vi "LVFunction_Imop_HAS file_GetInformation.vi"(0 "HAS file path":path, 11 "error in (no error)":errorcluster) -> (6 "HAS file information":T1 {"Source wavelength (nm)" format="%#_2g"}, 15 "error out":errorcluster)   [LabVIEW 2020]
doc: "Get informations from .has file.\n\n--------------------------------------------------------------------------------\n\n<B>has_file_pathIn</B> : Absolute path to the .has file.\n\n<B>has_file_pathOut</B> : Absolute path to the .has file.\n\n<B>haso_model</B> : Haso Sensor model.\n\n<B>haso_serial_number</B> : Haso Serial number.\n\n<B>revision</B> : Revision number.\n\n<B>size</B> : HasoData dimension (subpupil number)\n\n<B>step</B> : HasoData sampling step (um).\n\n<B>time_stamp</B> : Timestamp.\n\n<B>comments</B> : Comments\n\n<B>session_name</B> : Session name.\n\n<B>wavelength_nm</B> : Source wavelength (nm).\n\n<B>lower_calibration_wl</B> : Lower calibration wavelength (nm).\n\n<B>upper_calibration_wl</B> : Upper calibration wavelength (nm).\n\n<B>ErrorIn</B> : Error\n\n<B>ErrorOut</B> : Error"
uses:
  Controls/HAS File information.ctl
  Controls/General dimensions definition.ctl
  Controls/Point2D.ctl
  Controls/Point2Df.ctl
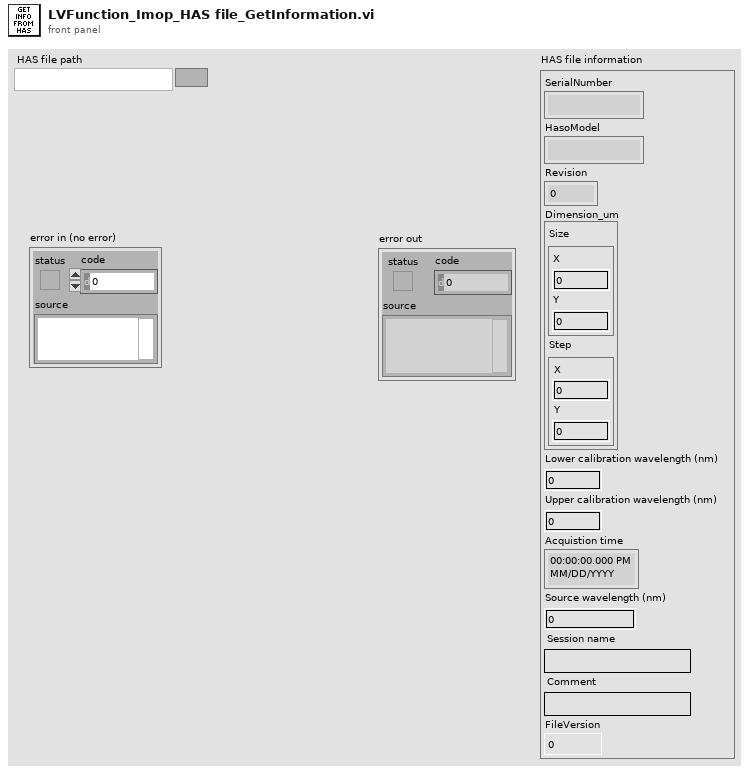
[diagram p1: front panel]
types:
  T1 = typedef "HAS File information.ctl" = cluster{"SerialNumber":string, "HasoModel":string, "Revision":u32, "Dimension_um":T2, "Lower calibration wavelength (nm)":dbl, "Upper calibration wavelength (nm)":dbl, "Acquistion time":timestamp, "Source wavelength (nm)":dbl, "Session name":string, "Comment":string, "FileVersion":i32}
  T2 = typedef "General dimensions definition.ctl" = cluster{"Size":T3, "Step":T4}
  T3 = typedef "Point2D.ctl" = cluster{"X":u32, "Y":u32}
  T4 = typedef "Point2Df.ctl" = cluster{"X":sgl, "Y":sgl}
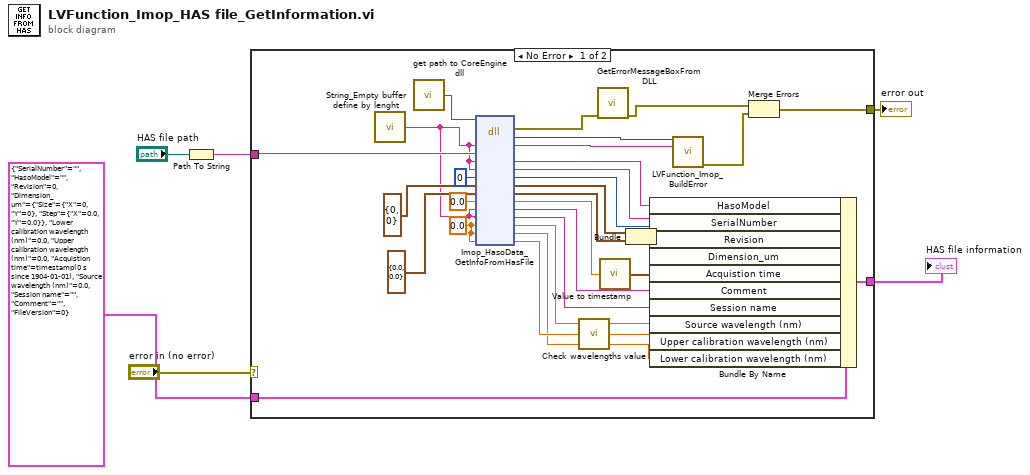
[diagram p0: block diagram]
diagram:
  n1 = Path To String(path="HAS file path") -> (string=w3:string)
  n2 = case shown="No Error" "error in (no error)" {
    selector: "error in (no error)" -> [_ w39]
    tunnel: [w17 w39] -> w5
    tunnel: w3 -> [w30 _]
    tunnel: T1 {"SerialNumber"="", "HasoModel"="", "Revision"=0, "Dimension_um"={"Size"={"X"=0, "Y"=0}, "Step"={"X"=0.0, "Y"=0.0}}, "Lower calibration wavelength (nm)"=0.0, "Upper calibration wavelength (nm)"=0.0, "Acquistion time"=timestamp(0 s since 1904-01-01), "Source wavelength (nm)"=0.0, "Session name"="", "Comment"="", "FileVersion"=0} ("HASO information 2") -> [w27 _]
    tunnel: [w23 _] -> w1
    frame No Error {
      w15 = 0.0 ("wavelength_nm")
      n3 = call "String_Empty buffer define by lenght.vi"() -> ("Empty buffer"=w16:string)  [unwired: 1 in]
      n4 = call "get path to CoreEngine dll.vi"() -> ("path to wavekit library"=w36:path)  [unwired: 14 in, 1 out]
      n5 = dll-call lib="D:/2_trunk/Soft_haso/ImOpCoreEngine4_LV2011/DLLs/ImopEngine4_vc100.dll" fn="Imop_HasoData_GetInfoFromHasFile"(path in=w36, "message"=w16, "HasFilePath"=w30, "HasoModel"=w16, "SerialNumber"=w16, "Revision"=u32 0, "size"=T3 {"X"=0, "Y"=0} ("Size"), "step"=T4 {"X"=0.0, "Y"=0.0} ("Step"), "TimeStamp"=0.0, "comment"=w16, "session_name"=w16, "wavelength_nm"=w15, "LowerCalibrationWl"=w15, "UpperCalibrationWl"=w15) -> (error out=w35:errorcluster, "return type"=w38:i32, "message"=w37:string, "HasoModel"=w26:string, "SerialNumber"=w25:string, "Revision"=w24:u32, "size"=w29:T3, "step"=w28:T4, "TimeStamp"=w13:dbl, "comment"=w20:string, "session_name"=w14:string, "wavelength_nm"=w12:dbl, "LowerCalibrationWl"=w10:dbl, "UpperCalibrationWl"=w11:dbl)  [unwired: 3 in, 1 out]
      n6 = call "Check wavelengths value.vi"("LowerCalibrationWl"=w10, "UpperCalibrationWl"=w11, "wavelength_nm"=w12) -> ("LowerCalibrationWl out"=w7:dbl, "UpperCalibrationWl out"=w8:dbl, "wavelength_nm out"=w9:dbl)
      n7 = call "GetErrorMessageBoxFromDLL.vi"("error IN"=w35) -> ("error OUT"=w19:errorcluster)  [unwired: 10 in]
      n8 = call "Value to timestamp.vi"("TimeStamp"=w13) -> ("Time Stamp"=w21:timestamp)
      n9 = Bundle("size"=w29, "step"=w28) -> (w22:cluster{"size":T3, "step":T4})  [unwired: 1 in]
      n10 = Bundle By Name(cluster=w27, "HasoModel"=w26, "SerialNumber"=w25, "Revision"=w24, "Dimension_um"=w22, "Acquistion time"=w21, "Comment"=w20, "Session name"=w14, "Source wavelength (nm)"=w9, "Upper calibration wavelength (nm)"=w8, "Lower calibration wavelength (nm)"=w7) -> (w23:T1)
      n11 = call "LVFunction_Imop_BuildError.vi"("code"=w38, "String to Prepend to source (\"\")"=w37) -> ("error out"=w18:errorcluster)  [unwired: 13 in]
      n12 = Merge Errors(w19, w18) -> (w17:errorcluster)
    }
    frame Error {
    }
  }
  "error out" <- w5
  "HAS file information" <- w1
